vi "Direction to string.vi"(11 "Direction":T1) -> (3 "Peak app":string)   [LabVIEW 2019, in "STAV lib.lvlib"]
uses:
  STAV lib.lvlib
  Param Direction.ctl
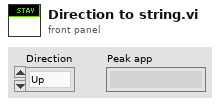
[diagram p1: front panel]
types:
  T1 = typedef "STAV lib.lvlib/Param Direction.ctl" = enum16{"Up", "Down", "Left", "Right"}
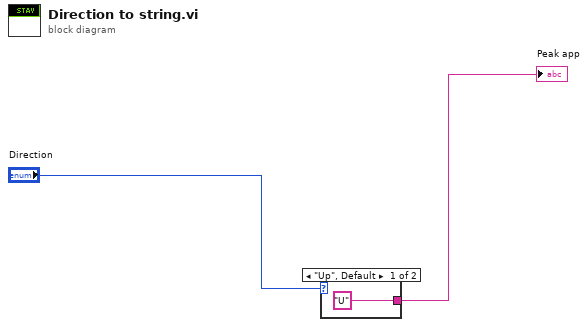
[diagram p0: block diagram]
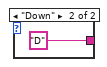
[diagram p2: hidden frame]
diagram:
  n1 = case shown="\"Up\", Default" "Direction" {
    tunnel: ["U" ("Peak app") "D" ("Peak app")] -> w2
    frame "Up", Default {
    }
    frame "Down" {
    }
  }
  "Peak app" <- w2
